vi "Update Entry.vi"(8 "Server":bool, 10 "Cluster":T4, 11 "TCP Network Connection in":refnum<k5>) -> (1 "Size":i32=1, 2 "Field Value Out":T1, 3 "Updated":bool)   [LabVIEW 2017]
uses:
  <vilib>/Rock Robotics/Network Tables/Field Data.ctl
  <vilib>/Rock Robotics/Network Tables/Field Type.ctl
  <vilib>/Rock Robotics/Network Tables/Sequence.ctl
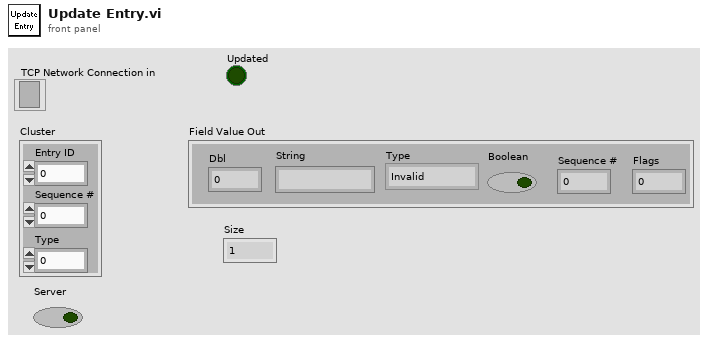
[diagram p1: front panel]
types:
  T1 = typedef "Field Data.ctl" = cluster{"Dbl":dbl, "String":string, "Type":T2, "Boolean":bool, "Sequence #":T3, "Flags":u8}
  T2 = typedef "Field Type.ctl" = enum8{"Invalid", "Bool", "Numeric", "String", "Raw", "Boolean Array", "Numeric Array", "String Array", "RPC"}
  T3 = typedef "Sequence.ctl" = u16
  T4 = cluster{"Entry ID":u16, "Sequence #":u16, "Type":u8}
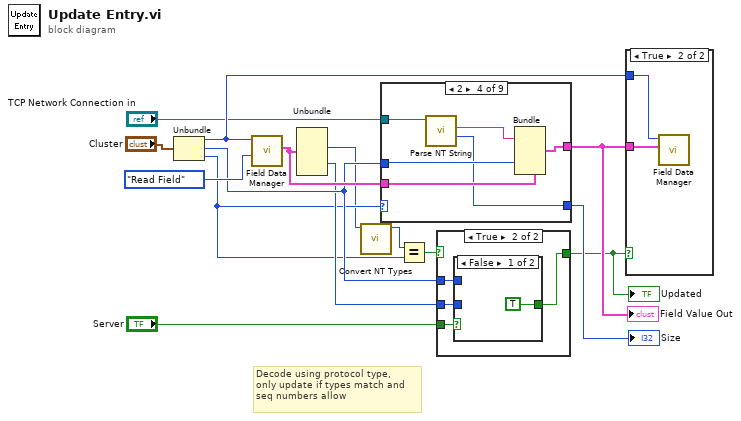
[diagram p0: block diagram]
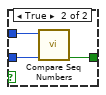
[diagram p3: hidden frame]
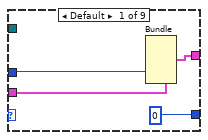
[diagram p5: hidden frame]
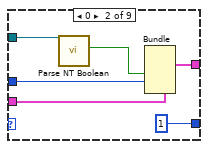
[diagram p6: hidden frame]
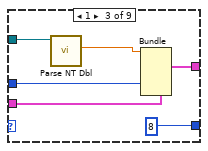
[diagram p7: hidden frame]
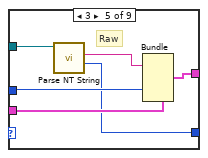
[diagram p8: hidden frame]
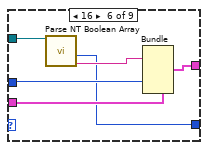
[diagram p9: hidden frame]
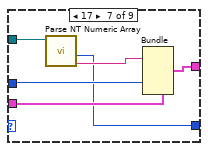
[diagram p10: hidden frame]
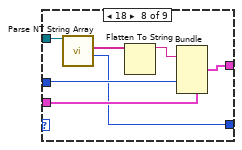
[diagram p11: hidden frame]
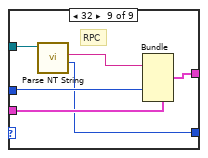
[diagram p12: hidden frame]
diagram:
  # "Decode using protocol type,\nonly update if types match and\nseq numbers allow"
  n1 = Unbundle("Cluster") -> ("Entry ID"=w15:u16, "Sequence #"=w6:u16, "Type"=w3:u8)
  n2 = call <vilib>:"Field Data Manager.vi"("Operation"=enum16{"Update Field", "Read Field"}."Read Field", "Field ID"=w15) -> ("Field Value Out"=w14:T1)  [unwired: 8 in, 1 out]
  n3 = Unbundle(w14) -> ("Type"=w2:T2, "Sequence #"=w5:T3)  [unwired: 4 out]
  n4 = call <vilib>:"Convert NT Types.vi"("Type in"=w2) -> ("Type out"=w1:u8)  [unwired: 10 in]
  n5 = case shown="2" w3 {
    tunnel: "TCP Network Connection in" -> [_ w22 w28 w34 w40 w46 w52 w59 w65]
    tunnel: w14 -> [w19 w23 w30 w36 w42 w48 w54 w61 w67]
    tunnel: [w18 w25 w31 w37 w43 w49 w55 w62 w68] -> w10
    tunnel: w6 -> [w17 w24 w29 w35 w41 w47 w53 w60 w66]
    tunnel: [0 1 8 w32 w38 w44 w50 w56 w63] -> w9
    frame Default {
      n6 = Bundle(cluster=w19, "Sequence #"=w17) -> (w18:T1)  [unwired: 5 in]
    }
    frame 0 {
      n7 = call <vilib>:"Parse NT Boolean.vi"("TCP Network Connection in"=w22) -> ("Boolean"=w21:bool)  [unwired: 9 in, 1 out]
      n8 = Bundle(cluster=w23, "Boolean"=w21, "Sequence #"=w24) -> (w25:T1)  [unwired: 4 in]
    }
    frame 1 {
      n9 = call <vilib>:"Parse NT Dbl.vi"("TCP Network Connection in"=w28) -> ("Double"=w27:dbl)  [unwired: 9 in, 1 out]
      n10 = Bundle(cluster=w30, "Dbl"=w27, "Sequence #"=w29) -> (w31:T1)  [unwired: 4 in]
    }
    frame 2 {
      n11 = call <vilib>:"Parse NT String.vi"("TCP Network Connection in"=w34) -> ("Size"=w32:i32, "String"=w33:string)  [unwired: 8 in, 1 out]
      n12 = Bundle(cluster=w36, "String"=w33, "Sequence #"=w35) -> (w37:T1)  [unwired: 4 in]
    }
    frame 3 {
      # "Raw"
      n13 = call <vilib>:"Parse NT String.vi"("TCP Network Connection in"=w40) -> ("Size"=w38:i32, "String"=w39:string)  [unwired: 8 in, 1 out]
      n14 = Bundle(cluster=w42, "String"=w39, "Sequence #"=w41) -> (w43:T1)  [unwired: 4 in]
    }
    frame 16 {
      n15 = call <vilib>:"Parse NT Boolean Array.vi"("TCP Network Connection in"=w46) -> ("String"=w45:string, "Size"=w44:i32)  [unwired: 7 in, 2 out]
      n16 = Bundle(cluster=w48, "String"=w45, "Sequence #"=w47) -> (w49:T1)  [unwired: 4 in]
    }
    frame 17 {
      n17 = call <vilib>:"Parse NT Numeric Array.vi"("TCP Network Connection in"=w52) -> ("String"=w51:string, "Size"=w50:i32)  [unwired: 7 in, 2 out]
      n18 = Bundle(cluster=w54, "String"=w51, "Sequence #"=w53) -> (w55:T1)  [unwired: 4 in]
    }
    frame 18 {
      n19 = call <vilib>:"Parse NT String Array.vi"("TCP Network Connection in"=w59) -> ("Size"=w56:i32, "String Array"=w58:string[])  [unwired: 8 in, 1 out]
      n20 = Flatten To String(anything=w58) -> (data string=w57:string)  [unwired: 3 in, 2 out]
      n21 = Bundle(cluster=w61, "String"=w57, "Sequence #"=w60) -> (w62:T1)  [unwired: 4 in]
    }
    frame 32 {
      # "RPC"
      n22 = call <vilib>:"Parse NT String.vi"("TCP Network Connection in"=w65) -> ("Size"=w63:i32, "String"=w64:string)  [unwired: 8 in, 1 out]
      n23 = Bundle(cluster=w67, "String"=w64, "Sequence #"=w66) -> (w68:T1)  [unwired: 4 in]
    }
  }
  "Field Value Out" <- w10
  "Size" <- w9
  n24 = Equal?(x=w1, y=w3) -> (x = y?=w4:bool)
  n25 = case shown="True" w4 {
    tunnel: [_ w72] -> w8
    tunnel: "Server" -> [_ w71]
    tunnel: w6 -> [_ w70]
    tunnel: w5 -> [_ w69]
    frame False {
    }
    frame True {
      n26 = case shown="False" w71 {
        tunnel: w70 -> [_ w76]
        tunnel: [TRUE ("A Greater Than B") w75] -> w72
        tunnel: w69 -> [_ w74]
        frame False {
        }
        frame True {
          n27 = call <vilib>:"Compare Seq Numbers.vi"("B"=w74, "A"=w76) -> ("A Greater Than B"=w75:bool)  [unwired: 8 in, 1 out]
        }
      }
    }
  }
  "Updated" <- w8
  n28 = case shown="True" w8 {
    tunnel: w15 -> [_ w78]
    tunnel: w10 -> [_ w77]
    frame False {
    }
    frame True {
      n29 = call <vilib>:"Field Data Manager.vi"("Field Value In"=w77, "Field ID"=w78) -> ()  [unwired: 8 in, 2 out]
    }
  }
